vi "Change update.vi"(8 "error in (no error)":errorcluster, 9 "Credit":dbl, 10 "Change":dbl, 11 "Dinero in":refnum<class "Dinero.lvclass">) -> (0 "error out":errorcluster, 3 "Dinero out":refnum<class "Dinero.lvclass">)   [LabVIEW 2020, in "Dinero.lvlib" / "Dinero.lvclass"]
uses:
  Dinero.lvclass
  <vilib>/ActorFramework/Actor/Actor.lvclass
  User Interface Messages/Get dinero Msg/Get dinero Msg.lvclass
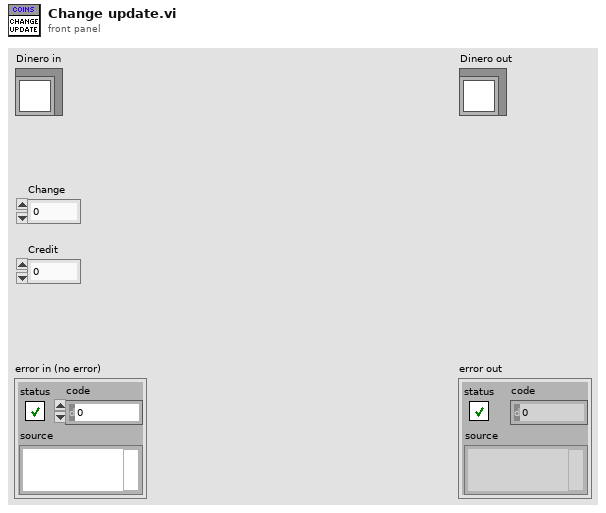
[diagram p1: front panel]
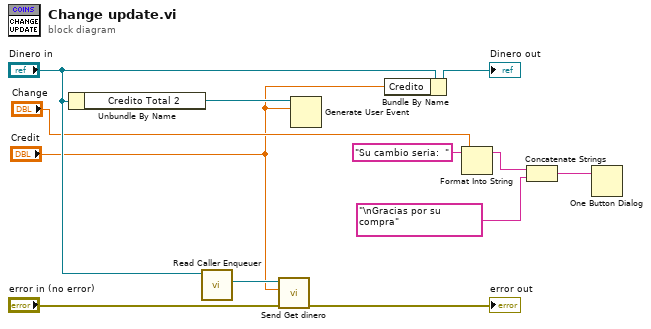
[diagram p0: block diagram]
diagram:
  n1 = Unbundle By Name("Dinero in") -> ("Credito Total 2"=w7:refnum<user-event>)
  n2 = call <vilib>:"Read Caller Enqueuer.vi"("Actor"="Dinero in") -> ("Caller Enqueuer"=w4:refnum<class "Message Enqueuer.lvclass">)  [unwired: 10 in]
  n3 = call "Send Get dinero.vi"("error in (no error)"="error in (no error)", "Dinero"="Credit", "Message Enqueuer"=w4) -> ("error out"=→"error out":errorcluster)  [unwired: 7 in, 1 out]
  n4 = Generate User Event(user event=w7, event data cluster="Credit") -> ()  [unwired: 2 in, 2 out]
  n5 = Bundle By Name(cluster="Dinero in", "Credito"="Credit") -> (→"Dinero out":refnum<class "Dinero.lvclass">)
  n6 = Format Into String(initial string="Su cambio seria:  ", "Change") -> (resulting string=w11:string)  [unwired: 2 in, 1 out]
  n7 = Concatenate Strings(w11, "\nGracias por su compra" ("string")) -> (w10:string)
  n8 = One Button Dialog(message=w10) -> ()  [unwired: 1 in, 1 out]
